vi "MCL Get Commanded Position.vi"(7 "handle":i32, 9 "zCom":dbl, 10 "yCom":dbl, 11 "xCom":dbl) -> (1 "zCom out":dbl, 2 "yCom out":dbl, 3 "xCom out":dbl, 5 "function return":i32)   [LabVIEW 2017, in "Madlib.lvlib"]
doc: "MADLIB_API int MCL_GetCommandedPosition(double *xCom, double *yCom, double *zCom, int handle);"
uses:
  Madlib.lvlib
  Madlib.dll
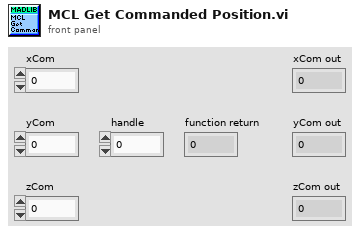
[diagram p1: front panel]
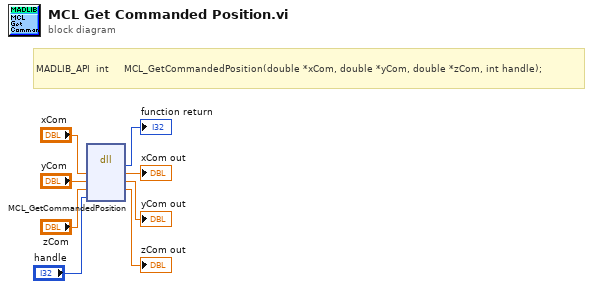
[diagram p0: block diagram]
diagram:
  # "MADLIB_API  int     MCL_GetCommandedPosition(double *xCom, double *yCom, double *zCom, int handle);"
  n1 = dll-call lib="C:/Users/francesco/dev/pump-probe/Piezo/lvlib/Madlib.*" fn="MCL_GetCommandedPosition"("xCom"="xCom", "yCom"="yCom", "zCom"="zCom", "handle"="handle") -> (→"function return":i32, "xCom"=→"xCom out":dbl, "yCom"=→"yCom out":dbl, "zCom"=→"zCom out":dbl)  [unwired: 4 in, 2 out]
